vi "ActionVIOnLoad.vi"(8 "error in":errorcluster, 11 "Device Item Ref in":T1 format="%.0x") -> (0 "error out":errorcluster, 3 "Device Item Ref out":T1 format="%.0x")   [LabVIEW 2020, in "Ballard MIL-STD-1553 System Explorer.lvlib" / "Implementation.lvlib"]
uses:
  Implementation.lvlib
  <vilib>/NI VeriStand/Custom Device API/Custom Device Item Ref.ctl
  NationalInstruments.VeriStand.SystemDefinitionAPI
  <vilib>/NI VeriStand/Custom Device API/Custom Device API.lvlib
  Scripting/Ballard MIL-STD-1553 Scripting.lvlib
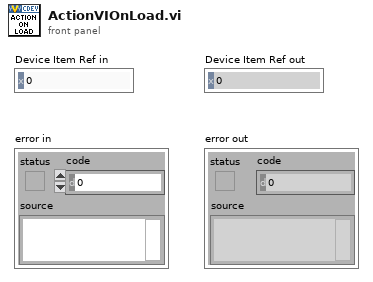
[diagram p1: front panel]
types:
  T1 = typedef "Custom Device API.lvlib/Custom Device Item Ref.ctl" = u64
  T2 = typedef "Custom Device API.lvlib/Custom Device Item Info.ctl" = cluster{"Name":string, "Is Channel":bool, "GUID":string, "Is Waveform":bool}
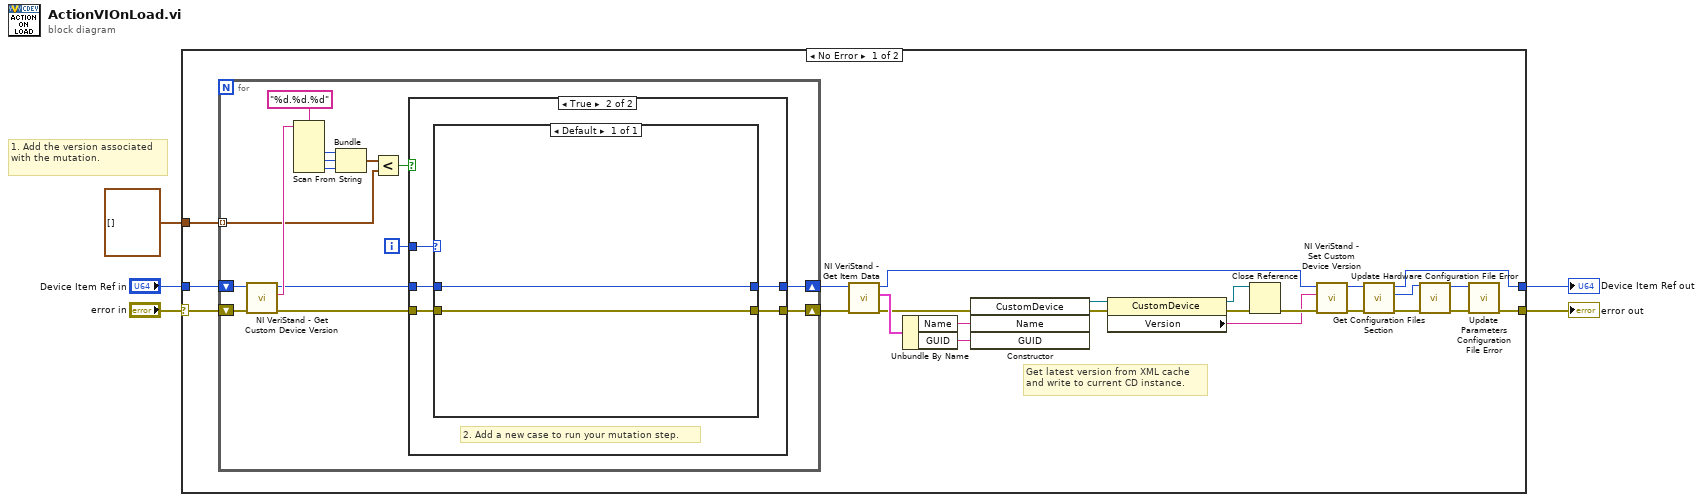
[diagram p0: block diagram]
diagram:
  # "1. Add the version associated with the mutation."
  n1 = case shown="No Error" "error in" {
    selector: "error in" -> [w29 w55]
    tunnel: [w7 w55] -> w3
    tunnel: "Device Item Ref in" -> [w28 w54]
    tunnel: [w6 w54] -> w2
    tunnel: cluster{i32, i32, i32}[] [] -> [w27 _]
    frame No Error {
      # "Get latest version from XML cache\nand write to current CD instance."
      n2 = for {
        shift-right: [w35] -> w25
        shift-left: w29 -> [w40]
        shift-right: [w33] -> w26
        shift-left: w28 -> [w39]
        tunnel: w27 -> [w30] mode=indexing
        i -> [w32]
        n3 = call <vilib>:"NI VeriStand - Get Custom Device Version.vi"("error in (no error)"=w40, "Device Ref in"=w39) -> ("error out"=w36:errorcluster, "Value"=w38:string, "Device Ref out"=w34:T1)  [unwired: 7 in]
        n4 = Scan From String(format string="%d.%d.%d", input string=w38) -> (output 1=w42:i32, output 2=w43:i32, output 3=w31:i32)  [unwired: 5 in, 3 out]
        n5 = Bundle(w42, w43, w31) -> (w44:cluster{i32, i32, i32})  [unwired: 1 in]
        n6 = Less?(x=w44, y=w30) -> (x < y?=w37:bool)
        n7 = case shown="True" w37 {
          tunnel: w36 -> [w46 w51]
          tunnel: [w46 w50] -> w35
          tunnel: w34 -> [w45 w47]
          tunnel: [w45 w48] -> w33
          tunnel: w32 -> [_ w49]
          frame False {
          }
          frame True {
            # "2. Add a new case to run your mutation step."
            n8 = case shown="Default" w49 {
              tunnel: w51 -> [w53]
              tunnel: [w53] -> w50
              tunnel: [w52] -> w48
              tunnel: w47 -> [w52]
              frame Default {
              }
            }
          }
        }
      }
      n9 = call <vilib>:"NI VeriStand - Get Item Data.vi"("error in (no error)"=w25, "Item Ref in"=w26) -> ("error out"=w21:errorcluster, "Item Info"=w24:T2, "Item Ref out"=w14:T1)  [unwired: 6 in, 1 out]
      n10 = Unbundle By Name(w24) -> ("Name"=w23:string, "GUID"=w22:string)
      n11 = constructor class="CustomDevice"(error in=w21, "Name"=w23, "GUID"=w22) -> (reference out=w20:refnum<k24>, error out=w19:errorcluster)  [unwired: 2 in, 3 out]
      n12 = property class="CustomDevice"(reference=w20, error in=w19) -> (reference out=w17:refnum<k24>, error out=w18:errorcluster, "Version"=w15:string)
      n13 = Close Reference(reference=w17, error in (no error)=w18) -> (error out=w16:errorcluster)
      n14 = call <vilib>:"NI VeriStand - Set Custom Device Version.vi"("error in (no error)"=w16, "Value"=w15, "Device Ref in"=w14) -> ("error out"=w12:errorcluster, "Device Ref out"=w13:T1)  [unwired: 7 in]
      n15 = call "Get Configuration Files Section.vi"("error in"=w12, "custom device in"=w13) -> ("error out"=w11:errorcluster, "configuration files section"=w10:T1, "custom device out"=w6:T1)  [unwired: 7 in]
      n16 = call "Update Hardware Configuration File Error.vi"("error in"=w11, "configuration files ref in"=w10) -> ("error out"=w8:errorcluster, "configuration files ref out"=w9:T1)  [unwired: 8 in]
      n17 = call "Update Parameters Configuration File Error.vi"("error in"=w8, "configuration files ref in"=w9) -> ("error out"=w7:errorcluster)  [unwired: 8 in, 1 out]
    }
    frame Error {
    }
  }
  "error out" <- w3
  "Device Item Ref out" <- w2
